vi "PQstatus.vi"(8 "error in (no error)":errorcluster, 10 "conn":u32) -> (0 "error out":errorcluster, 2 "PQStatus":T1(ring))   [LabVIEW 2018, in "libpqlv.lvlib"]
uses:
  libpqlv.lvlib
  lib/libpq.dll
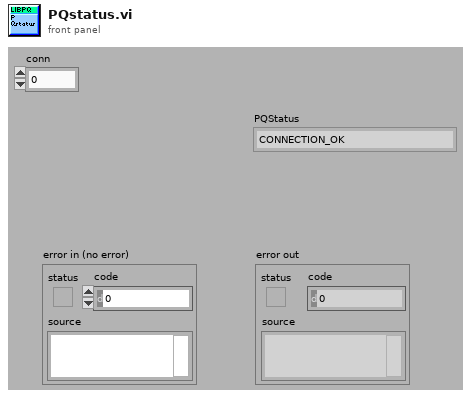
[diagram p1: front panel]
types:
  T1 = enum32{"CONNECTION_OK", "CONNECTION_BAD", "CONNECTION_STARTED", "CONNECTION_MADE", "CONNECTION_AWAITING_RESPONSE", "CONNECTION_AUTH_OK", "CONNECTION_SETENV", "CONNECTION_SSL_STARTUP", "CONNECTION_NEEDED"}
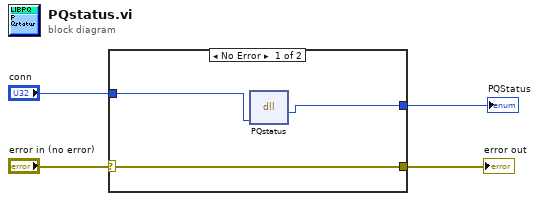
[diagram p0: block diagram]
diagram:
  n1 = case shown="No Error" "error in (no error)" {
    selector: "error in (no error)" -> [w7 w8]
    tunnel: [w7 w8] -> w3
    tunnel: [w6 _] -> w1
    tunnel: "conn" -> [w5 _]
    frame No Error {
      n2 = dll-call lib="C:/Users/ericsims/Documents/TC-3/DAQ/PostgreSQL2LabVIEW/libpqlv/lib/libpq.*" fn="PQstatus"("conn"=w5) -> ("PQstatus"=w6:u32)  [unwired: 4 in, 2 out]
    }
    frame Error {
    }
  }
  "error out" <- w3
  "PQStatus" <- w1
